vi "_LoadMassReference.vi"(4 "error in (no error)":errorcluster, 6 "Path":path, 7 "Polarity":enum32{"Positive", "Negative"}(radio)) -> (0 "error out":errorcluster, 3 "MassReference":cluster{"Mass":dbl, "Use":bool}[](array[cluster]))   [LabVIEW 2015]
uses:
  Type/_Log Command.ctl
  <vilib>/xml/Load XML File.vi
  <vilib>/xml/Close Reference(Node).vi
  <vilib>/xml/NI_XML.lvlib
  <resource>/objmgr/DOMUserDefRef.rc
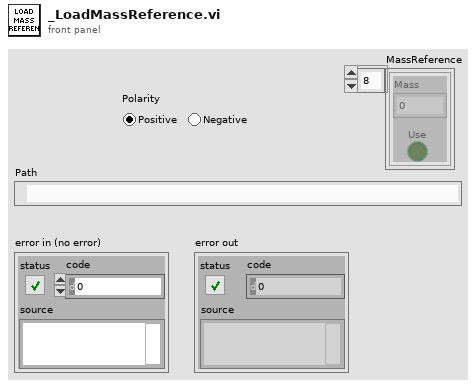
[diagram p1: front panel]
types:
  T1 = typedef "_Log Command.ctl" = enum16{"No Command", "Open", "Read", "Write", "Close", "Check Size"}
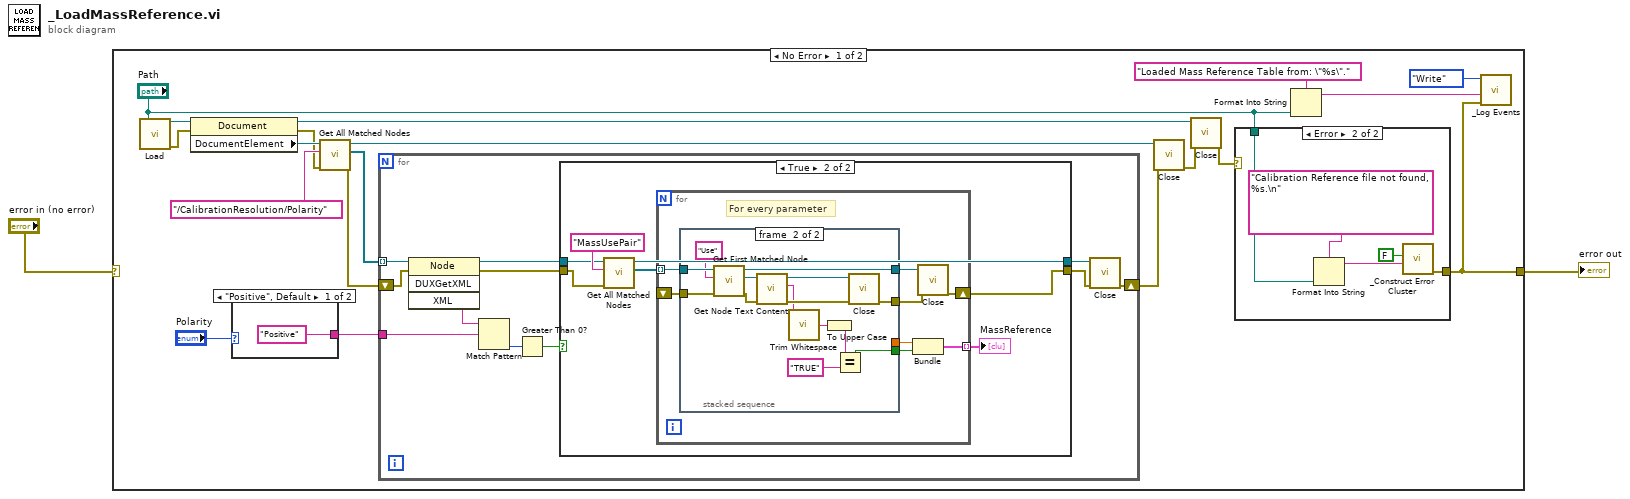
[diagram p0: block diagram]
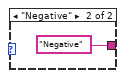
[diagram p3: hidden frame]
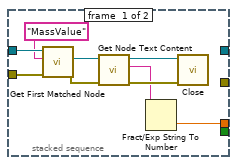
[diagram p5: hidden frame]
diagram:
  n1 = case shown="No Error" "error in (no error)" {
    selector: "error in (no error)" -> [_ w80]
    tunnel: [w3 w80] -> w2
    frame No Error {
      n2 = call-poly <vilib>:"Load.vi"("path to XML document"="Path") -> ("DOM document out"=w21:refnum<k20>, "error out"=w20:errorcluster)  [unwired: 12 in, 1 out]
      n3 = property on="Property Node" class="Document"(reference=w21, error in=w20) -> (reference out=w18:refnum<k20>, error out=w14:errorcluster, "DocumentElement"=w15:refnum<k20>)
      n4 = case shown="\"Positive\", Default" "Polarity" {
        tunnel: ["Positive" "Negative"] -> w9
        frame "Positive", Default {
        }
        frame "Negative" {
        }
      }
      n5 = call <vilib>:"Get All Matched Nodes.vi"("error in (no error)"=w14, "XPath expression"="/CalibrationResolution/Polarity", "node in"=w15) -> ("error out"=w12:errorcluster, "node result array"=w16:refnum<k20>[], "node out"=w13:refnum<k20>)  [unwired: 6 in]
      n6 = for {
        tunnel: w16 -> [w39] mode=indexing
        shift-right: [w37] -> w11
        shift-left: w12 -> [w38]
        tunnel: w9 -> [w35]
        n7 = invoke class="Node" method="DUXGetXML"(reference=w39, error in=w38) -> (reference out=w32:refnum<k20>, error out=w31:errorcluster, "XML"=w36:string)  [unwired: 2 in, 1 out]
        n8 = Match Pattern(string=w36, regular expression=w35) -> (offset past match=w34:i32)  [unwired: 1 in, 3 out]
        n9 = Greater Than 0?(x=w34) -> (x > 0?=w33:bool)
        n10 = case shown="True" w33 {
          tunnel: w32 -> [w41 w47]
          tunnel: w31 -> [w40 w46]
          tunnel: [w41 w45] -> w30
          tunnel: [w40 w43] -> w29
          frame False {
          }
          frame True {
            n11 = call <vilib>:"Get All Matched Nodes.vi"("error in (no error)"=w46, "XPath expression"="MassUsePair" ("regular expression"), "node in"=w47) -> ("node result array"=w44:refnum<k20>[], "node out"=w45:refnum<k20>)  [unwired: 6 in, 1 out]
            n12 = for {
              tunnel: w44 -> [w56] mode=indexing
              shift-right: [w54] -> w43
              shift-left: _ -> [w55]
              tunnel: [w49] -> w42 mode=indexing
              # "For every parameter"
              n13 = stacked-sequence {
                tunnel: w56 -> [w65 w79]
                tunnel: w55 -> [w64 w78]
                tunnel: [_ w76] -> w53
                tunnel: [_ w75] -> w52
                tunnel: [w57 _] -> w51
                tunnel: [_ w66] -> w50
                frame #0 {
                  n14 = call <vilib>:"Get First Matched Node.vi"("error in (no error)"=w64, "XPath expression"="MassValue", "node in"=w65) -> ("error out"=w59:errorcluster, "node result"=w62:refnum<k20>)  [unwired: 6 in, 1 out]
                  n15 = call <vilib>:"Get Node Text Content.vi"("error in (no error)"=w59, "node in"=w62) -> ("error out"=w60:errorcluster, "node text"=w58:string, "node out"=w61:refnum<k20>)  [unwired: 7 in]
                  n16 = Fract/Exp String To Number(string=w58) -> (number=w57:dbl)  [unwired: 3 in, 1 out]
                  n17 = call-poly <vilib>:"Close.vi"("error in (no error)"=w60, "node"=w61) -> ()  [unwired: 7 in, 1 out]
                }
                frame #1 {
                  n18 = call <vilib>:"Get First Matched Node.vi"("error in (no error)"=w78, "XPath expression"="Use", "node in"=w79) -> ("error out"=w73:errorcluster, "node result"=w74:refnum<k20>, "node out"=w76:refnum<k20>)  [unwired: 6 in]
                  n19 = call <vilib>:"Get Node Text Content.vi"("error in (no error)"=w73, "node in"=w74) -> ("error out"=w71:errorcluster, "node text"=w70:string, "node out"=w72:refnum<k20>)  [unwired: 7 in]
                  n20 = call <vilib>:"Trim Whitespace.vi"("string"=w70) -> ("trimmed string"=w69:string)  [unwired: 1 in]
                  n21 = To Upper Case(1:w69) -> (0:w68:string)
                  n22 = Equal?(x=w68, y="TRUE") -> (x = y?=w66:bool)
                  n23 = call-poly <vilib>:"Close.vi"("error in (no error)"=w71, "node"=w72) -> ("error out"=w75:errorcluster)  [unwired: 7 in]
                }
              }
              n24 = Bundle(w51, w50) -> (w49:cluster{dbl, bool})  [unwired: 1 in]
              n25 = call-poly <vilib>:"Close.vi"("error in (no error)"=w52, "node"=w53) -> ("error out"=w54:errorcluster)  [unwired: 7 in]
            }
            "MassReference" <- w42
          }
        }
        n26 = call-poly <vilib>:"Close.vi"("error in (no error)"=w29, "node"=w30) -> ("error out"=w37:errorcluster)  [unwired: 7 in]
      }
      n27 = call-poly <vilib>:"Close.vi"("error in (no error)"=w11, "node"=w13) -> ("error out"=w17:errorcluster)  [unwired: 7 in]
      n28 = call-poly <vilib>:"Close.vi"("error in (no error)"=w17, "node"=w18) -> ("error out"=w8:errorcluster)  [unwired: 7 in]
      n29 = case shown="Error" w8 {
        tunnel: "Path" -> [_ w24]
        tunnel: [_ w23] -> w3
        frame No Error {
        }
        frame Error {
          n30 = Format Into String(format string="Calibration Reference file not found, %s.\n", w24) -> (resulting string=w26:string)  [unwired: 2 in, 1 out]
          n31 = call "_Construct Error Cluster.vi"("reason"=w26, "CallingChain? (T)"=FALSE) -> ("error out"=w23:errorcluster)  [unwired: 5 in]
        }
      }
      n32 = Format Into String(format string="Loaded Mass Reference Table from: \"%s\".", "Path") -> (resulting string=w4:string)  [unwired: 2 in, 1 out]
      n33 = call "_Log Events.vi"("error in (no error)"=w3, "Event"=w4, "Log Command"=_Log_Command."Write" ("File Command")) -> ()  [unwired: 5 in, 2 out]
    }
    frame Error {
    }
  }
  "error out" <- w2
